vi "TPNT_DevInfo2Str.vi"(10 "Device In":T1={"device"="", "devupdate"=0.0, "next_update"=0, "devinterface"="", "TPs"=[], "Alarms"=TRUE, "monitor"=TRUE, "log sep"=""} {"TPs"."Log"."updaterate" format="%.2f"; "TPs"."Samples"."Values" format="%.2f"; "TPs"."Samples"."samples" min=1 step=1; "TPs"."Limits"."Nominal" format="%.2f"; "TPs"."Limits"."Upper" format="%.2f"; "TPs"."Limits"."Lower" format="%.2f"; "TPs"."update_rate" format="%.2f"; "devupdate" format="%.2f"}) -> (2 "TP out":string)   [LabVIEW 2016]
uses:
  TPNT_DeviceTPs.ctl
  TPNT_TP.ctl
  TPNT_Limits.ctl
  TPNT_Samples.ctl
  TPNT_Log.ctl
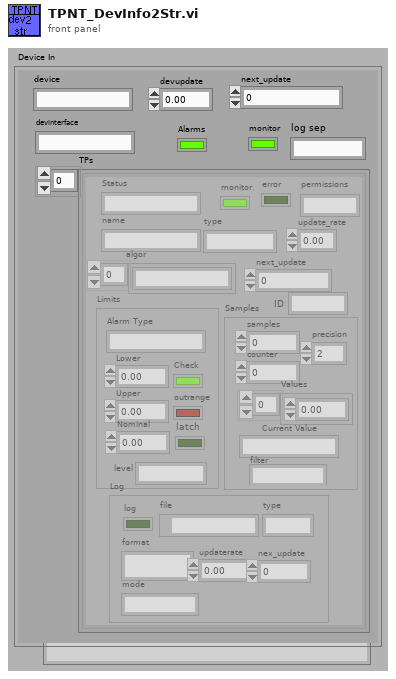
[diagram p1: front panel]
types:
  T1 = typedef "TPNT_DeviceTPs.ctl" = cluster{"device":string, "devupdate":dbl, "next_update":u32, "devinterface":string, "TPs":T2[], "Alarms":bool, "monitor":bool, "log sep":string}
  T2 = typedef "TPNT_TP.ctl" = cluster{"name":string, "type":string, "algor":string[], "update_rate":sgl, "Limits":T3, "Samples":T4, "next_update":u32, "Status":string, "monitor":bool, "error":bool, "Log":T5, "permissions":string, "ID":string}
  T3 = typedef "TPNT_Limits.ctl" = cluster{"Alarm Type":string, "Lower ":dbl, "Upper":dbl, "Nominal":dbl, "outrange":bool, "Check":bool, "latch":bool, "level":string}
  T4 = typedef "TPNT_Samples.ctl" = cluster{"samples":i32, "counter":i32, "Values":dbl[], "Current Value":string, "filter":string, "precision":u8}
  T5 = typedef "TPNT_Log.ctl" = cluster{"log":bool, "file":path, "type":string, "format":string, "updaterate":dbl, "nex_update":u32, "mode":string}
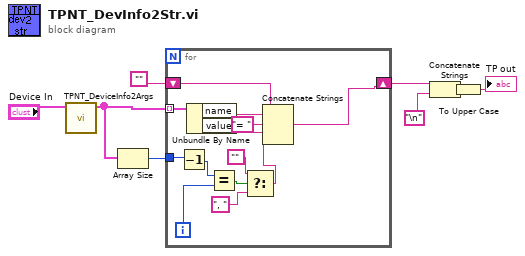
[diagram p0: block diagram]
diagram:
  n1 = call "TPNT_DeviceInfo2Args.vi"("Device IN"="Device In") -> ("values out"=w6:cluster{"name":string, "value":string}[])  [unwired: 10 out]
  n2 = Array Size(array=w6) -> (size(s)=w5:i32)
  n3 = for {
    tunnel: w6 -> [w21] mode=indexing
    shift-right: [w12] -> w4
    shift-left: "" -> [w19]
    tunnel: w5 -> [w18]
    i -> [w16]
    n4 = Decrement(x=w18) -> (x-1=w17:i32)
    n5 = Unbundle By Name(w21) -> ("name"=w20:string, "value"=w10:string)
    n6 = Equal?(x=w17, y=w16) -> (x = y?=w15:bool)
    n7 = Select(t="", s=w15, f=", ") -> (s? t:f=w9:string)
    n8 = Concatenate Strings(w19, w20, "= " ("string"), w10, w9) -> (w12:string)
  }
  n9 = Concatenate Strings(w4, "\n") -> (w2:string)
  n10 = To Upper Case(1:w2) -> (0:→"TP out":string)
